vi "ROI coord bundler.vi"(8 "error in (no error)":errorcluster, 11 "Experiment folder path":path) -> (0 "error out":errorcluster, 1 "ROI Attributes":T1[](array[typedef]) {"ROI group ID" format="%#_6f"; "Laser Power (%)" format="%#_6f"; "Zoom" format="%#_6f"; "Frame Size" format="%#_6f"; "Number of lines" format="%#_6f"; "Composite ID" format="%#_6f"; "Angle (deg)" format="%#_6f"; "ROI Time (ns)" format="%#_6f"; "ROI ID" format="%#_6f"; "Pixels in ROI" format="%#_6f"; "ROI index" format="%#_6f"; "Z stop" format="%#_6f"; "Y stop" format="%#_6f"; "X stop" format="%#_6f"; "Z start" format="%#_6f"; "X start" format="%#_6f"; "Y start" format="%#_6f"}, 2 "Total number of miniscans":i32, 3 "ROI Coordinates (broken down to miniscans)":T2, 4 "ROI Attributes (broken down to miniscans)":T1[](array[typedef]) {"ROI group ID" format="%#_6f"; "Laser Power (%)" format="%#_6f"; "Zoom" format="%#_6f"; "Frame Size" format="%#_6f"; "Number of lines" format="%#_6f"; "Composite ID" format="%#_6f"; "Angle (deg)" format="%#_6f"; "ROI Time (ns)" format="%#_6f"; "ROI ID" format="%#_6f"; "Pixels in ROI" format="%#_6f"; "ROI index" format="%#_6f"; "Z stop" format="%#_6f"; "Y stop" format="%#_6f"; "X stop" format="%#_6f"; "Z start" format="%#_6f"; "X start" format="%#_6f"; "Y start" format="%#_6f"}, 5 "Number of pixels in single miniscan":i32, 6 "Zoom":dbl[](array[numeric]), 7 "Number of POIs":i32)   [LabVIEW 2013]
uses:
  User Interface/Visualisation/Functional Imaging Viewer/Typedefs/ROI parameters data type.ctl
  Typedefs/ROI XY coordinates cluster.ctl
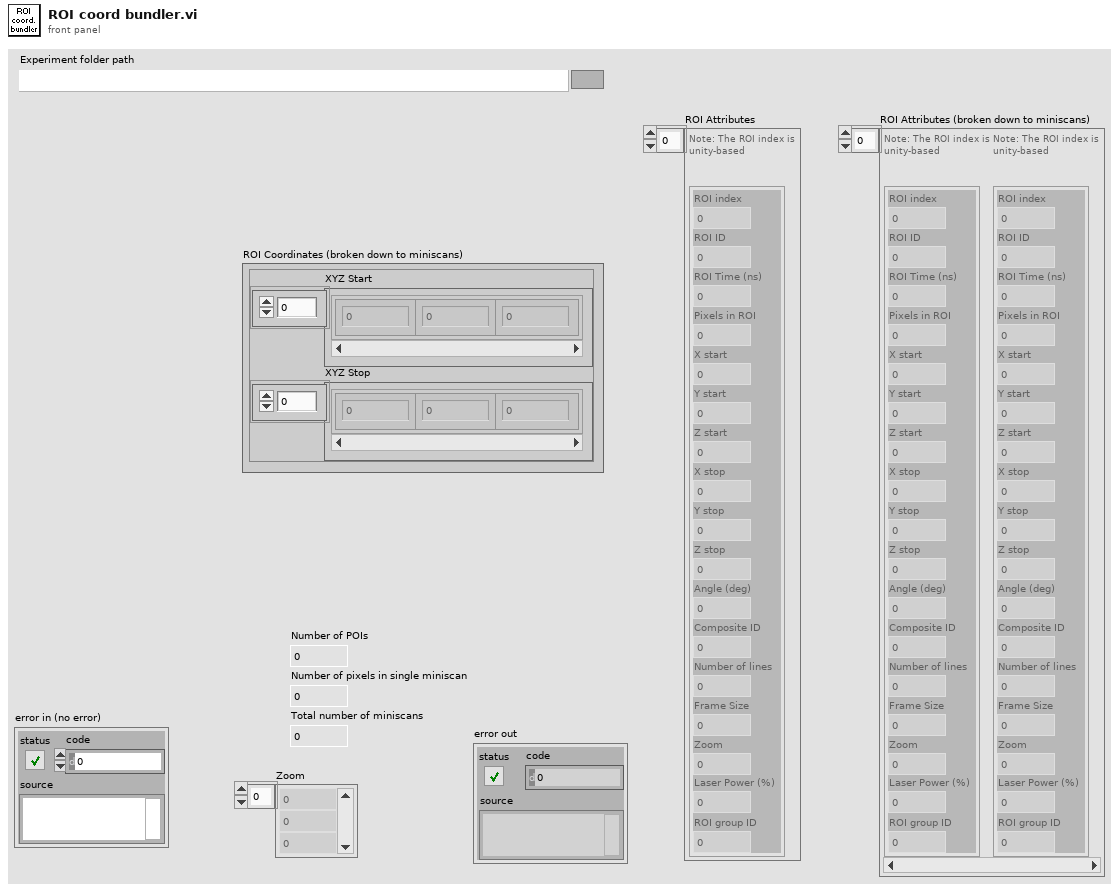
[diagram p1: front panel]
types:
  T1 = typedef "ROI parameters data type.ctl" = cluster{"ROI index":dbl, "ROI ID":dbl, "ROI Time (ns)":dbl, "Pixels in ROI":dbl, "X start":dbl, "Y start":dbl, "Z start":dbl, "X stop":dbl, "Y stop":dbl, "Z stop":dbl, "Angle (deg)":dbl, "Composite ID":dbl, "Number of lines":dbl, "Frame Size":dbl, "Zoom":dbl, "Laser Power (%)":dbl, "ROI group ID":dbl}
  T2 = typedef "ROI XY coordinates cluster.ctl" = cluster{"XYZ Start":cluster{"X":sgl, "Y":sgl, "Z":sgl}[], "XYZ Stop":cluster{"X":sgl, "Y":sgl, "Z":sgl}[]}
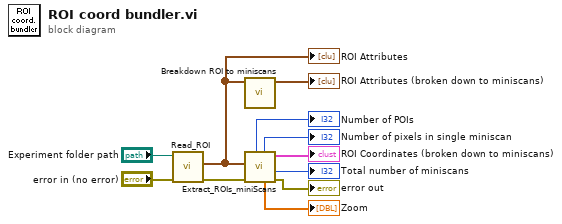
[diagram p0: block diagram]
diagram:
  n1 = call "Read_ROI.vi"("error in"="error in (no error)", "Experiment folder path"="Experiment folder path") -> ("error out"=w9:errorcluster, "ROI setup"=w2:T1[])  [unwired: 8 in]
  "ROI Attributes" <- w2
  n2 = call "Breakdown ROI to miniscans.vi"("ROI Attributes"=w2) -> ("ROI Attributes (broken down to miniscans)"=→"ROI Attributes (broken down to miniscans)":T1[])  [unwired: 10 in]
  n3 = call "Extract_ROIs_miniScans.vi"("error in (no error)"=w9, "ROI Attributes"=w2) -> ("error out"=→"error out":errorcluster, "Total number of miniscans"=→"Total number of miniscans":i32, "ROI Coordinates (broken down to miniscans)"=→"ROI Coordinates (broken down to miniscans)":T2, "Zoom"=→"Zoom":dbl[], "Number of pixels in single X miniscan"=→"Number of pixels in single miniscan":i32, "number of POI"=→"Number of POIs":i32)  [unwired: 2 in, 2 out]
